vi "Untitled 1 (SubVI).vi"(9 "X":dbl, 10 "Y":dbl) -> (1 "Roll":dbl, 2 "Hover":bool, 3 "Pitch":dbl)   [LabVIEW 2014]
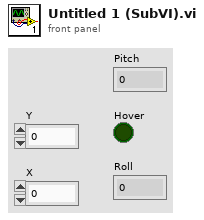
[diagram p1: front panel]
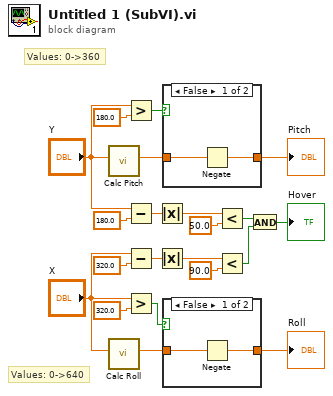
[diagram p0: block diagram]
diagram:
  # "Values: 0->640"
  # "Values: 0->360"
  n1 = call "Calc Pitch.vi"("Position"="Y") -> ("Pitch"=w15:dbl)  [unwired: 10 in]
  n2 = call "Calc Roll.vi"("Position"="X") -> ("Roll"=w16:dbl)  [unwired: 10 in]
  n3 = Greater?(x="Y", y=180.0) -> (0:w12:bool)
  n4 = Subtract(x="Y", y=180.0) -> (x-y=w4:dbl)
  n5 = Subtract(x="X", y=320.0) -> (x-y=w17:dbl)
  n6 = Greater?(x="X", y=320.0) -> (0:w14:bool)
  n7 = Absolute Value(x=w4) -> (abs(x)=w6:dbl)
  n8 = Absolute Value(x=w17) -> (abs(x)=w19:dbl)
  n9 = case shown="False" w12 {
    tunnel: w15 -> [w23 w24]
    tunnel: [w22 w24] -> w10
    frame False {
      n10 = Negate(x=w23) -> (-x=w22:dbl)
    }
    frame True {
    }
  }
  "Pitch" <- w10
  n11 = case shown="False" w14 {
    tunnel: w16 -> [w26 w27]
    tunnel: [w25 w27] -> w9
    frame False {
      n12 = Negate(x=w26) -> (-x=w25:dbl)
    }
    frame True {
    }
  }
  "Roll" <- w9
  n13 = Less?(x=w6, y=50.0) -> (x < y?=w2:bool)
  n14 = Less?(x=w19, y=90.0) -> (x < y?=w1:bool)
  n15 = And(x=w2, y=w1) -> (x .and. y?=→"Hover":bool)
